vi "ShutDown.vi"(8 "error in (no error)":errorcluster, 11 "FolloWin in":refnum<class "FolloWin.lvclass">) -> (0 "error out":errorcluster)   [LabVIEW 2023, in "FolloWin.lvclass"]
doc: "ShutsDown the Object"
uses:
  FolloWin.lvclass
  FolloWin.lvclass/FolloWin.ctl
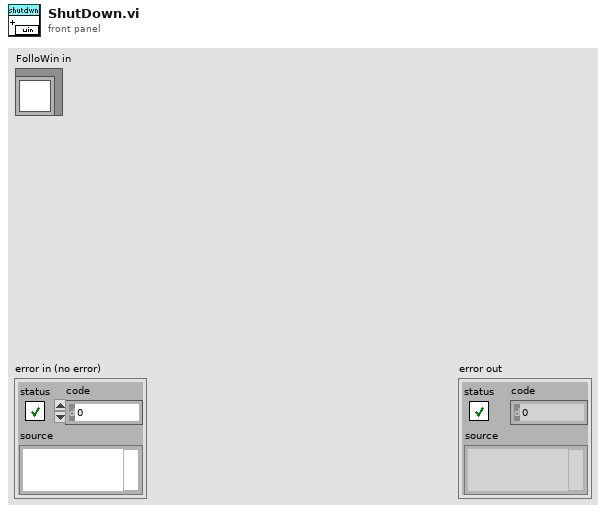
[diagram p1: front panel]
types:
  T1 = enum32{"Bad", "Idle", "Run top level", "Running"}
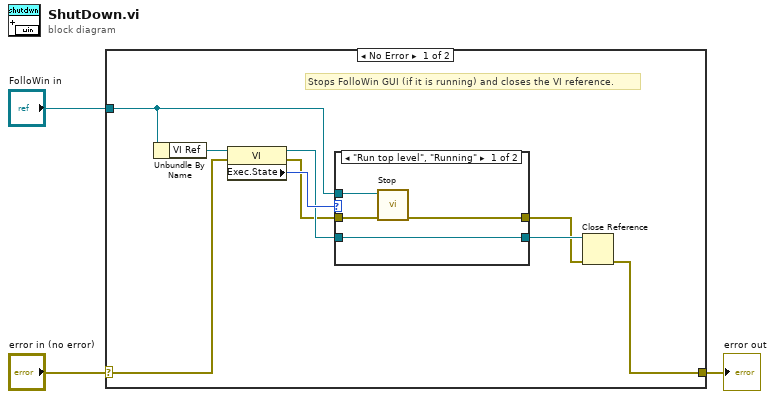
[diagram p0: block diagram]
diagram:
  n1 = case shown="No Error" "error in (no error)" {
    selector: "error in (no error)" -> [w5 w19]
    tunnel: [w6 w19] -> w2
    tunnel: "FolloWin in" -> [w9 _]
    frame No Error {
      # "Stops FolloWin GUI (if it is running) and closes the VI reference."
      n2 = Unbundle By Name(w9) -> ("VI Ref"=w12:refnum<vi>)
      n3 = property on="Property Node" class="VI"(reference=w12, error in=w5) -> (reference out=w10:refnum<vi>, error out=w4:errorcluster, "Exec.State"=w11:T1)
      n4 = case shown="\"Run top level\", \"Running\"" w11 {
        tunnel: w10 -> [w13 w17]
        tunnel: w9 -> [w16 _]
        tunnel: w4 -> [w15 w18]
        tunnel: [w14 w18] -> w7
        tunnel: [w13 w17] -> w8
        frame "Run top level", "Running" {
          n5 = call-dynamic "Stop.vi"("error in (no error)"=w15, "FolloWin in"=w16) -> ("error out"=w14:errorcluster)  [unwired: 8 in, 1 out]
        }
        frame Default {
        }
      }
      n6 = Close Reference(reference=w8, error in (no error)=w7) -> (error out=w6:errorcluster)
    }
    frame Error {
    }
  }
  "error out" <- w2
